vi "LOG tbl (SubVI).vi"(7 "t [s]":dbl, 8 "outer cmd [deg]":T1, 9 "middle cmd [deg]":T2, 10 "inner cmd [deg]":T1, 11 "MonitorBlock":dbl[](array[numeric])) -> (1 "ACCEL":cluster{dbl, dbl, dbl} {"?" format="%1_6g"}, 2 "RATE":cluster{dbl, dbl, dbl} {"?" format="%1_6g"}, 3 "POS":cluster{dbl, dbl, dbl} {"?" format="%_6g"; "?" format="%#1_6g"})   [LabVIEW 2017]
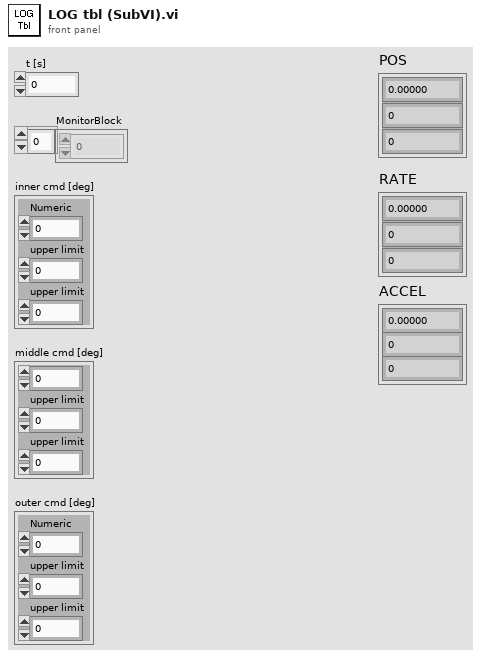
[diagram p1: front panel]
types:
  T1 = cluster{"Numeric":dbl, "upper limit":dbl, "upper limit":dbl}
  T2 = cluster{dbl, "upper limit":dbl, "upper limit":dbl}
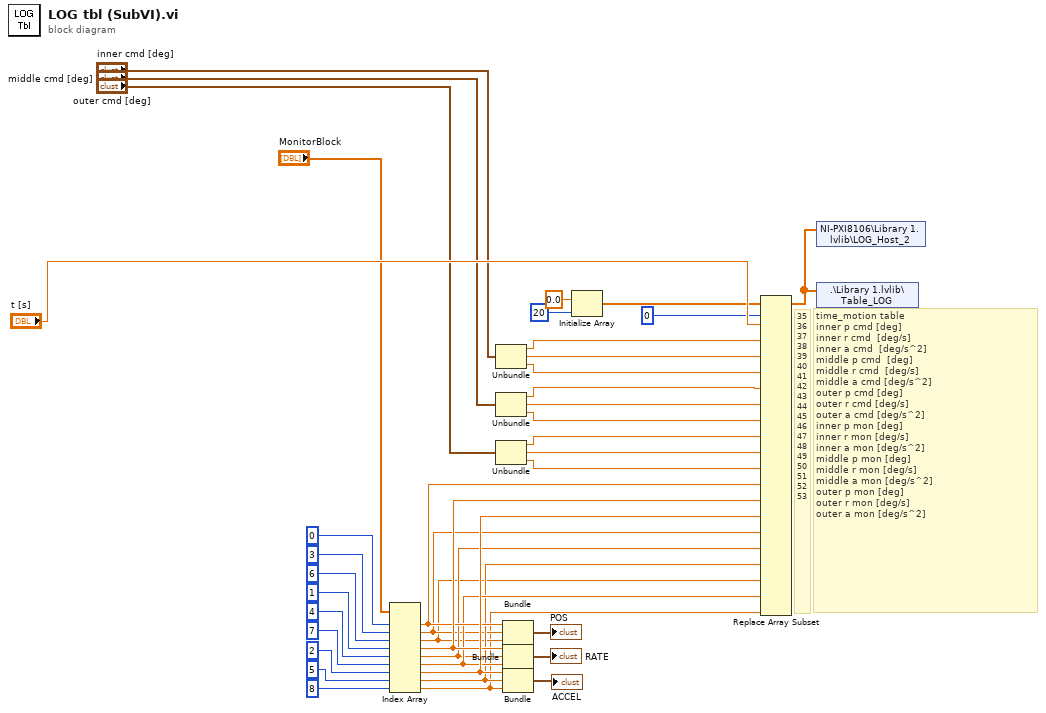
[diagram p0: block diagram]
diagram:
  # "time_motion table\ninner p cmd [deg]\ninner r cmd  [deg/s]\ninner a cmd  [deg/s^2]\nmiddle p cmd  [deg]\nmiddle r cmd  [deg/s]\nmiddle a cmd [deg/s^2]\nouter p cmd [deg]\nouter r cmd [deg/s]\nouter a cmd [deg/s^2]\ninner p mon [deg]\ninner r mon [deg/s]\ninner a mon [deg/s^2]\nmiddle p mon [deg]\nmiddle r mon [deg/s]\nmiddle a mon [deg/s^2]\nouter p mon [deg]\nouter r mon [deg/s]\nouter a mon [deg/s^2]"
  # "35\n36\n37\n38\n39\n40\n41\n42\n43\n44\n45\n46\n47\n48\n49\n50\n51\n52\n53"
  n1 = Index Array(array="MonitorBlock", index #1=0 ("index"), index #2=3 ("index"), index #3=6 ("index"), index #4=1 ("index"), index #5=4 ("index"), index #6=7 ("index"), index #7=2 ("index"), index #8=5 ("index"), index #9=8 ("index")) -> (element #1=w36:dbl, element #2=w29:dbl, element #3=w28:dbl, element #4=w37:dbl, element #5=w30:dbl, element #6=w32:dbl, element #7=w39:dbl, element #8=w31:dbl, element #9=w18:dbl)
  n2 = Unbundle("inner cmd [deg]") -> ("Numeric"=w26:dbl, "upper limit"=w19:dbl, "upper limit"=w20:dbl)
  n3 = Unbundle("middle cmd [deg]") -> (w27:dbl, "upper limit"=w21:dbl, "upper limit"=w22:dbl)
  n4 = Unbundle("outer cmd [deg]") -> ("Numeric"=w25:dbl, "upper limit"=w23:dbl, "upper limit"=w24:dbl)
  n5 = Bundle(w36, w29, w28) -> (→"POS":cluster{dbl, dbl, dbl})  [unwired: 1 in]
  n6 = Bundle(w37, w30, w32) -> (→"RATE":cluster{dbl, dbl, dbl})  [unwired: 1 in]
  n7 = Bundle(w39, w31, w18) -> (→"ACCEL":cluster{dbl, dbl, dbl})  [unwired: 1 in]
  n8 = Initialize Array(0.0 ("element"), 20 ("dimension size")) -> (w16:dbl[])
  n9 = Replace Array Subset(array=w16, new element #1="t [s]", index #1=0 ("index"), new element #2=w26, new element #3=w19, new element #4=w20, new element #5=w27, new element #6=w21, new element #7=w22, new element #8=w25, new element #9=w23, new element #10=w24, new element #11=w36, new element #12=w37, new element #13=w39, new element #14=w29, new element #15=w30, new element #16=w31, new element #17=w28, new element #18=w32, new element #19=w18) -> (w38:dbl[])  [unwired: 18 in]
  n10 = shared-variable "NI-PXI8106\\Library 1.lvlib\\LOG_Host_2"(w38) -> ()  [unwired: 1 in, 1 out]
  n11 = shared-variable ".\\Library 1.lvlib\\Table_LOG"(w38) -> ()  [unwired: 1 in, 1 out]
